vi "Enable-Disable UI Tab Ctrls.vi"(7 "Array":T1(array[ring]), 8 "error in (no error)":errorcluster, 10 "Tab Ctrl In":refnum<vi>) -> (0 "error out":errorcluster)   [LabVIEW 2023]
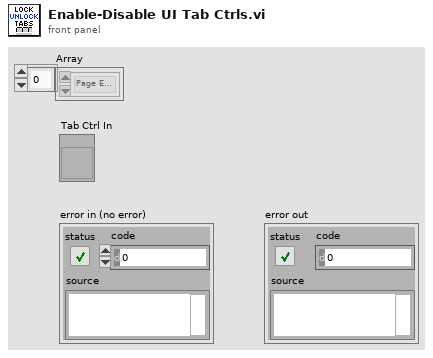
[diagram p1: front panel]
types:
  T1 = enum32{"Page Enabled", "Page Disabled", "Page Disabled & Grayed"}[]
  T2 = enum8{"Enabled", "Disabled", "Disabled and Grayed Out"}
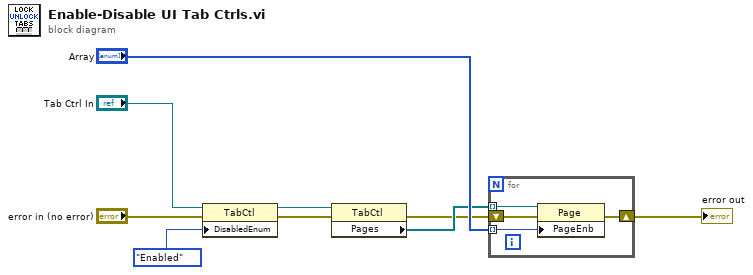
[diagram p0: block diagram]
diagram:
  n1 = property class="TabCtl"(reference="Tab Ctrl In", error in="error in (no error)", "DisabledEnum"=T2."Enabled" ("Disabled")) -> (reference out=w3:refnum<vi>, error out=w2:errorcluster)
  n2 = property class="TabCtl"(reference=w3, error in=w2) -> (error out=w4:errorcluster, "Pages"=w5:refnum<vi>[])  [unwired: 1 out]
  n3 = for {
    shift-right: [w13] -> w8
    shift-left: w4 -> [w12]
    tunnel: w5 -> [w11] mode=indexing
    tunnel: "Array" -> [w10] mode=indexing
    n4 = property class="Page"(reference=w11, error in=w12, "PageEnb"=w10) -> (error out=w13:errorcluster)  [unwired: 1 out]
  }
  "error out" <- w8
